vi "Compute 1D Index.vi"(1 "Size(s)":u32[](array[numeric]), 2 "Indices":u32[](array[numeric])) -> (0 "1D Index":i32)   [LabVIEW 2012, in "TD Tools.lvlib"]
uses:
  TD Tools.lvlib
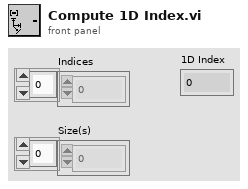
[diagram p1: front panel]
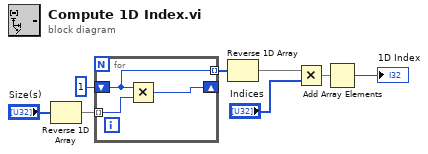
[diagram p0: block diagram]
diagram:
  n1 = Reverse 1D Array(array="Size(s)") -> (reversed array=w6:u32[])
  n2 = for {
    shift-right: [w10] -> _
    shift-left: 1 ("Index") -> [w9]
    tunnel: w6 -> [w11] mode=indexing
    tunnel: [w9] -> w7 mode=indexing
    n3 = Multiply(x=w9, y=w11) -> (x*y=w10:u32)
  }
  n4 = Reverse 1D Array(array=w7) -> (reversed array=w8:u32[])
  n5 = Multiply(x=w8, y="Indices") -> (x*y=w2:u32[])
  n6 = Add Array Elements(numeric array=w2) -> (sum=→"1D Index":u32)
